vi "Test.vi"() -> ()   [LabVIEW 2009]
panel:
  out "port":u16
  out "unsigned byte array 2":u8[](array[numeric])
  out "name":string
  in  "stop":bool
  out "unsigned byte array":u8[](array[numeric])
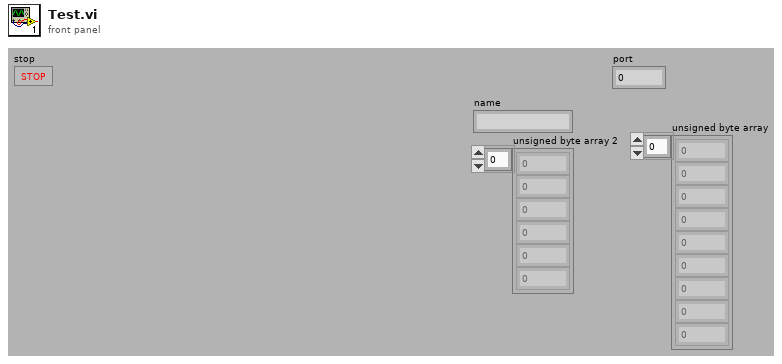
[diagram p1: front panel]
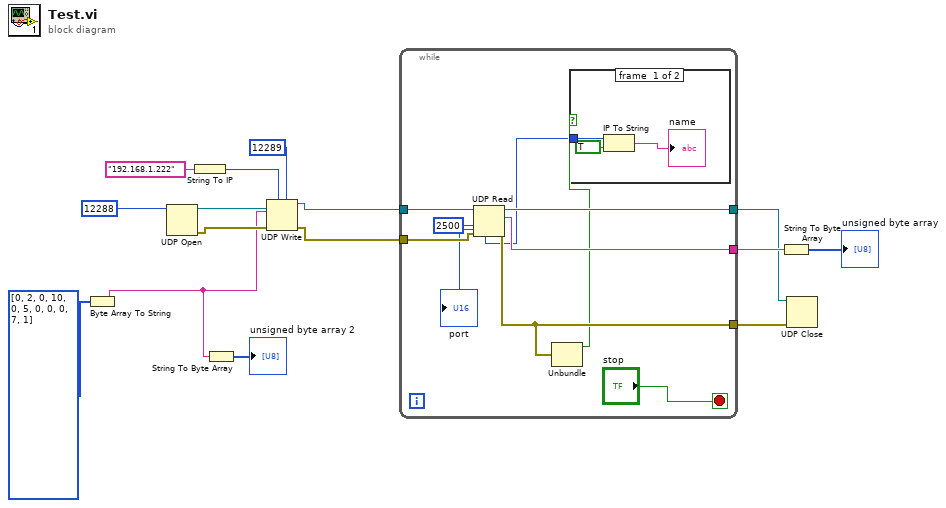
[diagram p0: block diagram]
diagram:
  n1 = Byte Array To String(unsigned byte array=u8[] [0, 2, 0, 10, 0, 5, 0, 0, 0, 7, 1]) -> (string=w4:string)
  n2 = UDP Open(11:u16 12288 ("port")) -> (port=w15:refnum<k16>, 0:w10:errorcluster)  [unwired: 4 in, 1 out]
  n3 = String To IP(1:"192.168.1.222" ("name")) -> (0:w1:u32)
  n4 = String To Byte Array(string=w4) -> (unsigned byte array=→"unsigned byte array 2":u8[])
  n5 = UDP Write(address=w1, port or service name=u16 12289, connection ID=w15, data in=w4, 8:w10) -> (error out=w9:errorcluster, 3:w11:refnum<k16>)  [unwired: 1 in]
  n6 = while {
    tunnel: w11 -> [w25]
    tunnel: w9 -> [w23]
    tunnel: [w22] -> w8
    tunnel: [w21] -> w6
    tunnel: [w20] -> w5
    stop <- "stop" stop-if-true
    n7 = UDP Read(connection ID=w25, timeout ms (25000)=2500, 8:w23) -> (data out=w22:string, error out=w20:errorcluster, 3:w21:refnum<k16>, 4:→"port":u16, 6:w18:u32)  [unwired: 1 in]
    n8 = Unbundle(w20) -> ("status"=w19:bool)  [unwired: 2 out]
    n9 = case shown="True" w19 {
      tunnel: w18 -> [w27 _]
      frame #0 {
        n10 = IP To String(1:TRUE ("dot notation? (F)"), 2:w27) -> (0:→"name":string)
      }
      frame #1 {
      }
    }
  }
  n11 = String To Byte Array(string=w8) -> (unsigned byte array=→"unsigned byte array":u8[])
  n12 = UDP Close(connection ID=w6, 8:w5) -> ()  [unwired: 2 out]
